vi "PDF_Interface_PDF Protokoll EPA1065_InterferenceVerification.vi"(8 "error in (no error)":errorcluster caption="Fehler (Eingang, kein Fehler)", 11 "Save PDF File Path":path) -> (0 "error out":errorcluster caption="Fehler (Ausgang)")   [LabVIEW 2020, in "EPA 1065.lvlib" / "Interference verificaton 1065-375.lvlib"]
uses:
  Interference verificaton 1065-375.lvlib
  Visualisierungs Elemente/String - Ausgabefeld.ctl
  ResultTable.ctl
  Sprachverwaltung/FGV Aktion Tabelle zerlegen.ctl
  <vilib>/Utility/miscctls.llb/LVRowAndColumnTypeDef.ctl
  Aktion FGV Interference.ctl
  Seiten/FT-IR/FGV FT-IR Aktionen.ctl
  Aktion Index uebersetzten.ctl
  Seiten/System Einstellungen V2/Aktioen FGV System Konstanten.ctl
  PDF_Interface/PDF Protokoll Standard Kopf Optionen.ctl
  <vilib>/Simplicity AI/SAI_PDF_API/Classes/Context/Controls/SAI_PDF_PDF Details.ctl
  PDF_Interface/PDF Interface Helper/PDFContentType.ctl
  PDF_Interface/PDF Interface Helper/PDFTableContentType.ctl
  PDF_Interface/PDF Interface Helper/PDFResults.ctl
  PDF_Interface/PDF Interface Helper/PDFResultPictures.ctl
  PDF_Interface/PDF Interface Helper/PDFCommentPosition.ctl
  PDF_Interface/PDF Interface Helper/PDFPageBreak.ctl
  PDF_Interface/PDF Interface Helper/PDFTablePictures.ctl
  PDF_Interface/PDF Interface Helper/PDFBemerkung.ctl
  <vilib>/Simplicity AI/SAI_PDF_API/Classes/Context/Controls/SAI_PDF_Text Align.ctl
  <vilib>/Simplicity AI/SAI_PDF_API/Classes/Context/Controls/SAI_PDF_Font.ctl
  <vilib>/Simplicity AI/SAI_PDF_API/Classes/Context/Controls/SAI_PDF_Font Encoding.ctl
  Allgemein/allgemeine Sub-VIs.lvlib
  Seiten/FT-IR/Span/Spanfaktor.lvlib
  Seiten/FT-IR/FT-IR.lvlib
  Sprachverwaltung/Sprachverwaltung.lvlib
  Seiten/System Einstellungen V2/System Einstellungen V2.lvlib
  PDF_Interface/PDF Interface.lvlib
  PDF_Interface/PDF Interface Helper/PDF Interface Helper.lvlib
  <vilib>/Simplicity AI/SAI_PDF_API/Classes/Context/Context.lvclass
  Linearisierung V2/Protokoll/Protokoll.lvlib
panel:
  out "[ppm]":sgl=1.0 caption="Grenze:" min=0 format="%#.6g"
  out "[ppm]":sgl=120.0 caption="Querempfindlichkeit:" min=0 format="%#.6g"
  out "LIN Ausgabetabelle":T1
  out "Komponente:":T2 caption="ppm"
  out "ErgebnisTabelle":string[][](table) caption="Tabelle 3"
  out "Header Tabelle":string[][](table) caption="Tabelle"
  # "Interference Verification - EPA § 1065.375"
  # "Ergebnis"
  # "Analysis"
  # "Komponente:"
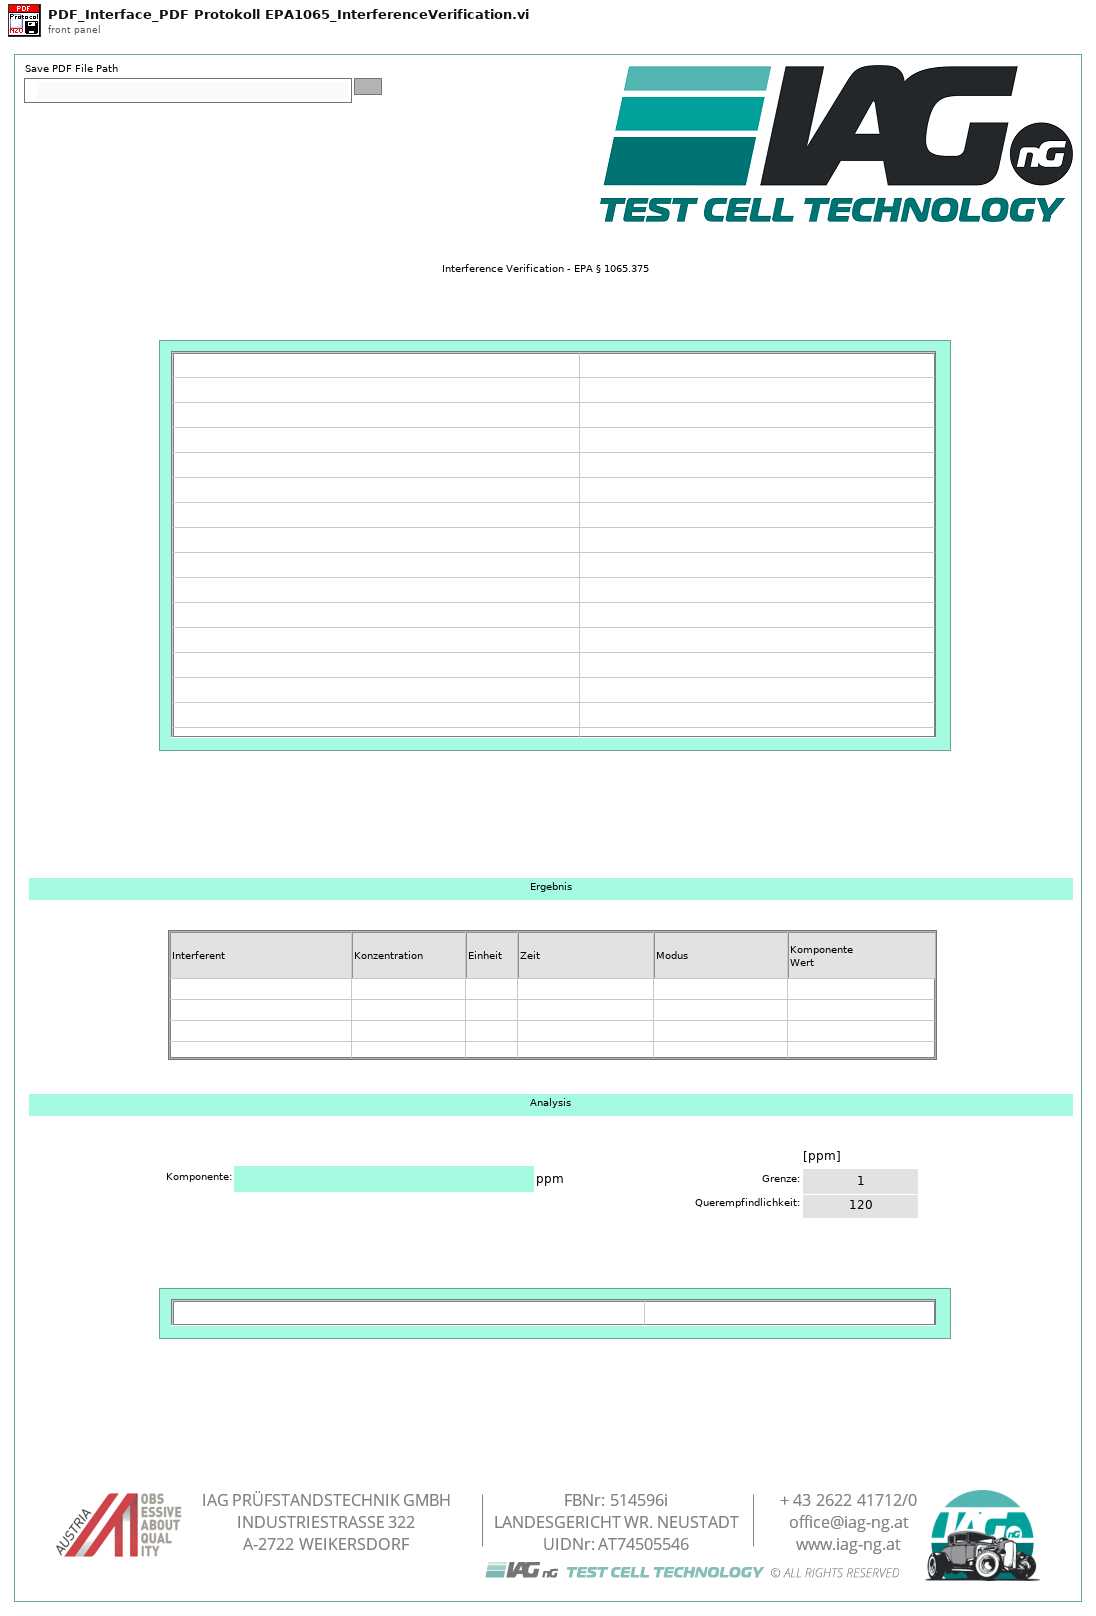
[diagram p1: front panel]
types:
  T1 = typedef "EPA 1065.lvlib/Interference verificaton 1065-375.lvlib/ResultTable.ctl" = string[][]
  T2 = typedef "String - Ausgabefeld.ctl" = string
  T3 = typedef "Sprachverwaltung.lvlib/FGV Aktion Tabelle zerlegen.ctl" = enum16{"laden", "vereinzeln", "speichern"}
  T4 = typedef "PDF Interface.lvlib/PDF Protokoll Standard Kopf Optionen.ctl" = cluster{"Analysator":bool, "FT-IR Rezept":bool, "Gasteiler":bool, "Gas Komponente":bool, "Gas Flasche":bool, "LIN Protokoll":bool, "Operator":bool}
  T5 = typedef "System Einstellungen V2.lvlib/Aktioen FGV System Konstanten.ctl" = enum16{"lesen", "laden", "speichern", "Sprache"}
  T6 = typedef "EPA 1065.lvlib/Interference verificaton 1065-375.lvlib/Aktion Index uebersetzten.ctl" = enum16{"lesen", "schreiben", "auswerten"}
  T7 = typedef "FT-IR.lvlib/FGV FT-IR Aktionen.ctl" = enum16{"lesen", "NOG setzen", "NOS setzen", "Initialisieren", "speichern", "ALLES setzen", "FT-IR Spektrum loggen", "Komm Stoppen", "Spektrum LogKonfig"}
  T8 = typedef "EPA 1065.lvlib/Interference verificaton 1065-375.lvlib/Aktion FGV Interference.ctl" = enum16{"Lesen", "TestKonfig", "TestSetting", "Einheiten", "Ergebnis", "Laden", "Tabelle", "Speichern", "löschen"}
  T9 = typedef "LVRowAndColumnTypeDef.ctl" = cluster{"Row":i32, "Column":i32}
  T10 = typedef "PDF Interface.lvlib/PDF Interface Helper.lvlib/PDFResults.ctl" = cluster{"Results":cluster{"Result Text":string, "Result":bool}[], "ResultPictures":T11, "use Pictures":bool, "Image Scale (%)":sgl, "Autoscale? (T)":bool, "Horizontal Align":i32, "Position":i32}
  T11 = typedef "PDF Interface.lvlib/PDF Interface Helper.lvlib/PDFResultPictures.ctl" = cluster{"Yes Ctl Refnum":refnum<vi>, "No Ctl Refnum":refnum<vi>}
  T12 = typedef "PDF Interface.lvlib/PDF Interface Helper.lvlib/PDFContentType.ctl" = cluster{"Titel":string, "Header Table":string[][], "Table Array":T13[], "Bemerkungen":T17[]}
  T13 = typedef "PDF Interface.lvlib/PDF Interface Helper.lvlib/PDFTableContentType.ctl" = cluster{"TableHeader":string[], "Table":string[][], "Relative Column Widths (%)":sgl[], "Results":T10, "PositionBemerkung":T14, "PageBreak":T15, "TablePictures":T16, "Horizontal Align":i32}
  T14 = typedef "PDF Interface.lvlib/PDF Interface Helper.lvlib/PDFCommentPosition.ctl" = enum16{"before", "after"}
  T15 = typedef "PDF Interface.lvlib/PDF Interface Helper.lvlib/PDFPageBreak.ctl" = enum16{"none", "before", "after", "after comment"}
  T16 = typedef "PDF Interface.lvlib/PDF Interface Helper.lvlib/PDFTablePictures.ctl" = cluster{"Ctl Refnum In":refnum<vi>[], "RowOrColumn":enum16{"Row", "Column"}, "IndexToInsert":u16, "Image Scale (%)":sgl[], "Autoscale? (T)":bool[], "Horizontal Align":i32}
  T17 = typedef "PDF Interface.lvlib/PDF Interface Helper.lvlib/PDFBemerkung.ctl" = cluster{"Bemerkung Text":string, "Align (Left)":T18, "Add Line Feeds (F:No)":bool, "Font":T19}
  T18 = typedef "SAI_PDF_Toolkit.lvlib/Context.lvclass/SAI_PDF_Text Align.ctl" = i32
  T19 = typedef "SAI_PDF_Toolkit.lvlib/Context.lvclass/SAI_PDF_Font.ctl" = cluster{"Font":string, "Size":i32, "Colour":u32, "Bold":bool, "Italic":bool, "Underline":bool, "Strikethrough":bool, "Font Encoding":T20}
  T20 = typedef "SAI_PDF_Toolkit.lvlib/Context.lvclass/SAI_PDF_Font Encoding.ctl" = enum16{"Cp1252, WinANSI", "IdentityH", "IdentityV", "Cp1250", "Cp1257", "MacRoman"}
  T21 = typedef "SAI_PDF_Toolkit.lvlib/Context.lvclass/SAI_PDF_PDF Details.ctl" = cluster{"Title":string, "Subject":string, "Keywords":string, "Author":string, "Creator":string}
  T22 = cluster{"Header Footer Text Cluster":cluster{"Header Text":string, "Footer Text":string, "Time":string, "Page Number":string}, "PDF Details":T21}
  T23 = typedef "EPA 1065.lvlib/Interference verificaton 1065-375.lvlib/TestSetting.ctl" = cluster{"Bearbeiter:":string, "Pfad:":path, "Textname:":string, "Analysator":T24}
  T24 = typedef "System Einstellungen V2.lvlib/Analysatoren.ctl" = string
  T25 = typedef "EPA 1065.lvlib/Interference verificaton 1065-375.lvlib/TestKonfig.ctl" = cluster{"Komponente:":u16, "Modus":T26, "CG Aufschaltzeit:":dbl, "Interferent 1:":u16, "Interferent 2:":u16, "Interferent 3:":u16, "Gasflaschen Nr.:":string, "Gasflaschen Nr.: 2":string, "Gasflaschen Nr.: 3":string, "Inter 1 aktiv":bool, "Inter 2 aktiv":bool, "Inter 3 aktiv":bool, "Accuracy":string, "Accuracy 2":string, "Accuracy 3":string, "Konzentration 1:":dbl, "Konzentration 2:":dbl, "Konzentration 3:":dbl}
  T26 = typedef "EPA 1065.lvlib/Interference verificaton 1065-375.lvlib/Modus.ctl" = u16
  T27 = typedef "EPA 1065.lvlib/Interference verificaton 1065-375.lvlib/Komponenten.ctl" = cluster{"Komponente":T2, "Komponente Index":i32, "Komponente 2":T2, "Komponente Index 2":i32, "Komponente 3":T2, "Komponente Index 3":i32, "Interferent 1":T2, "Interferent Index":i32, "Interferent 2":T2, "Interferent 2 Index":i32, "Interferent 3":T2, "Interferent 3 Index":i32, "Interferent 4":T2, "Interferent 4 Index":i32}
  T28 = cluster{"Modell":string, "ProjektNummer":string, "Software Version":string, "Seriennummer":string}
  T29 = cluster{"Header Size":i32, "Column Ratio left":sgl[]}
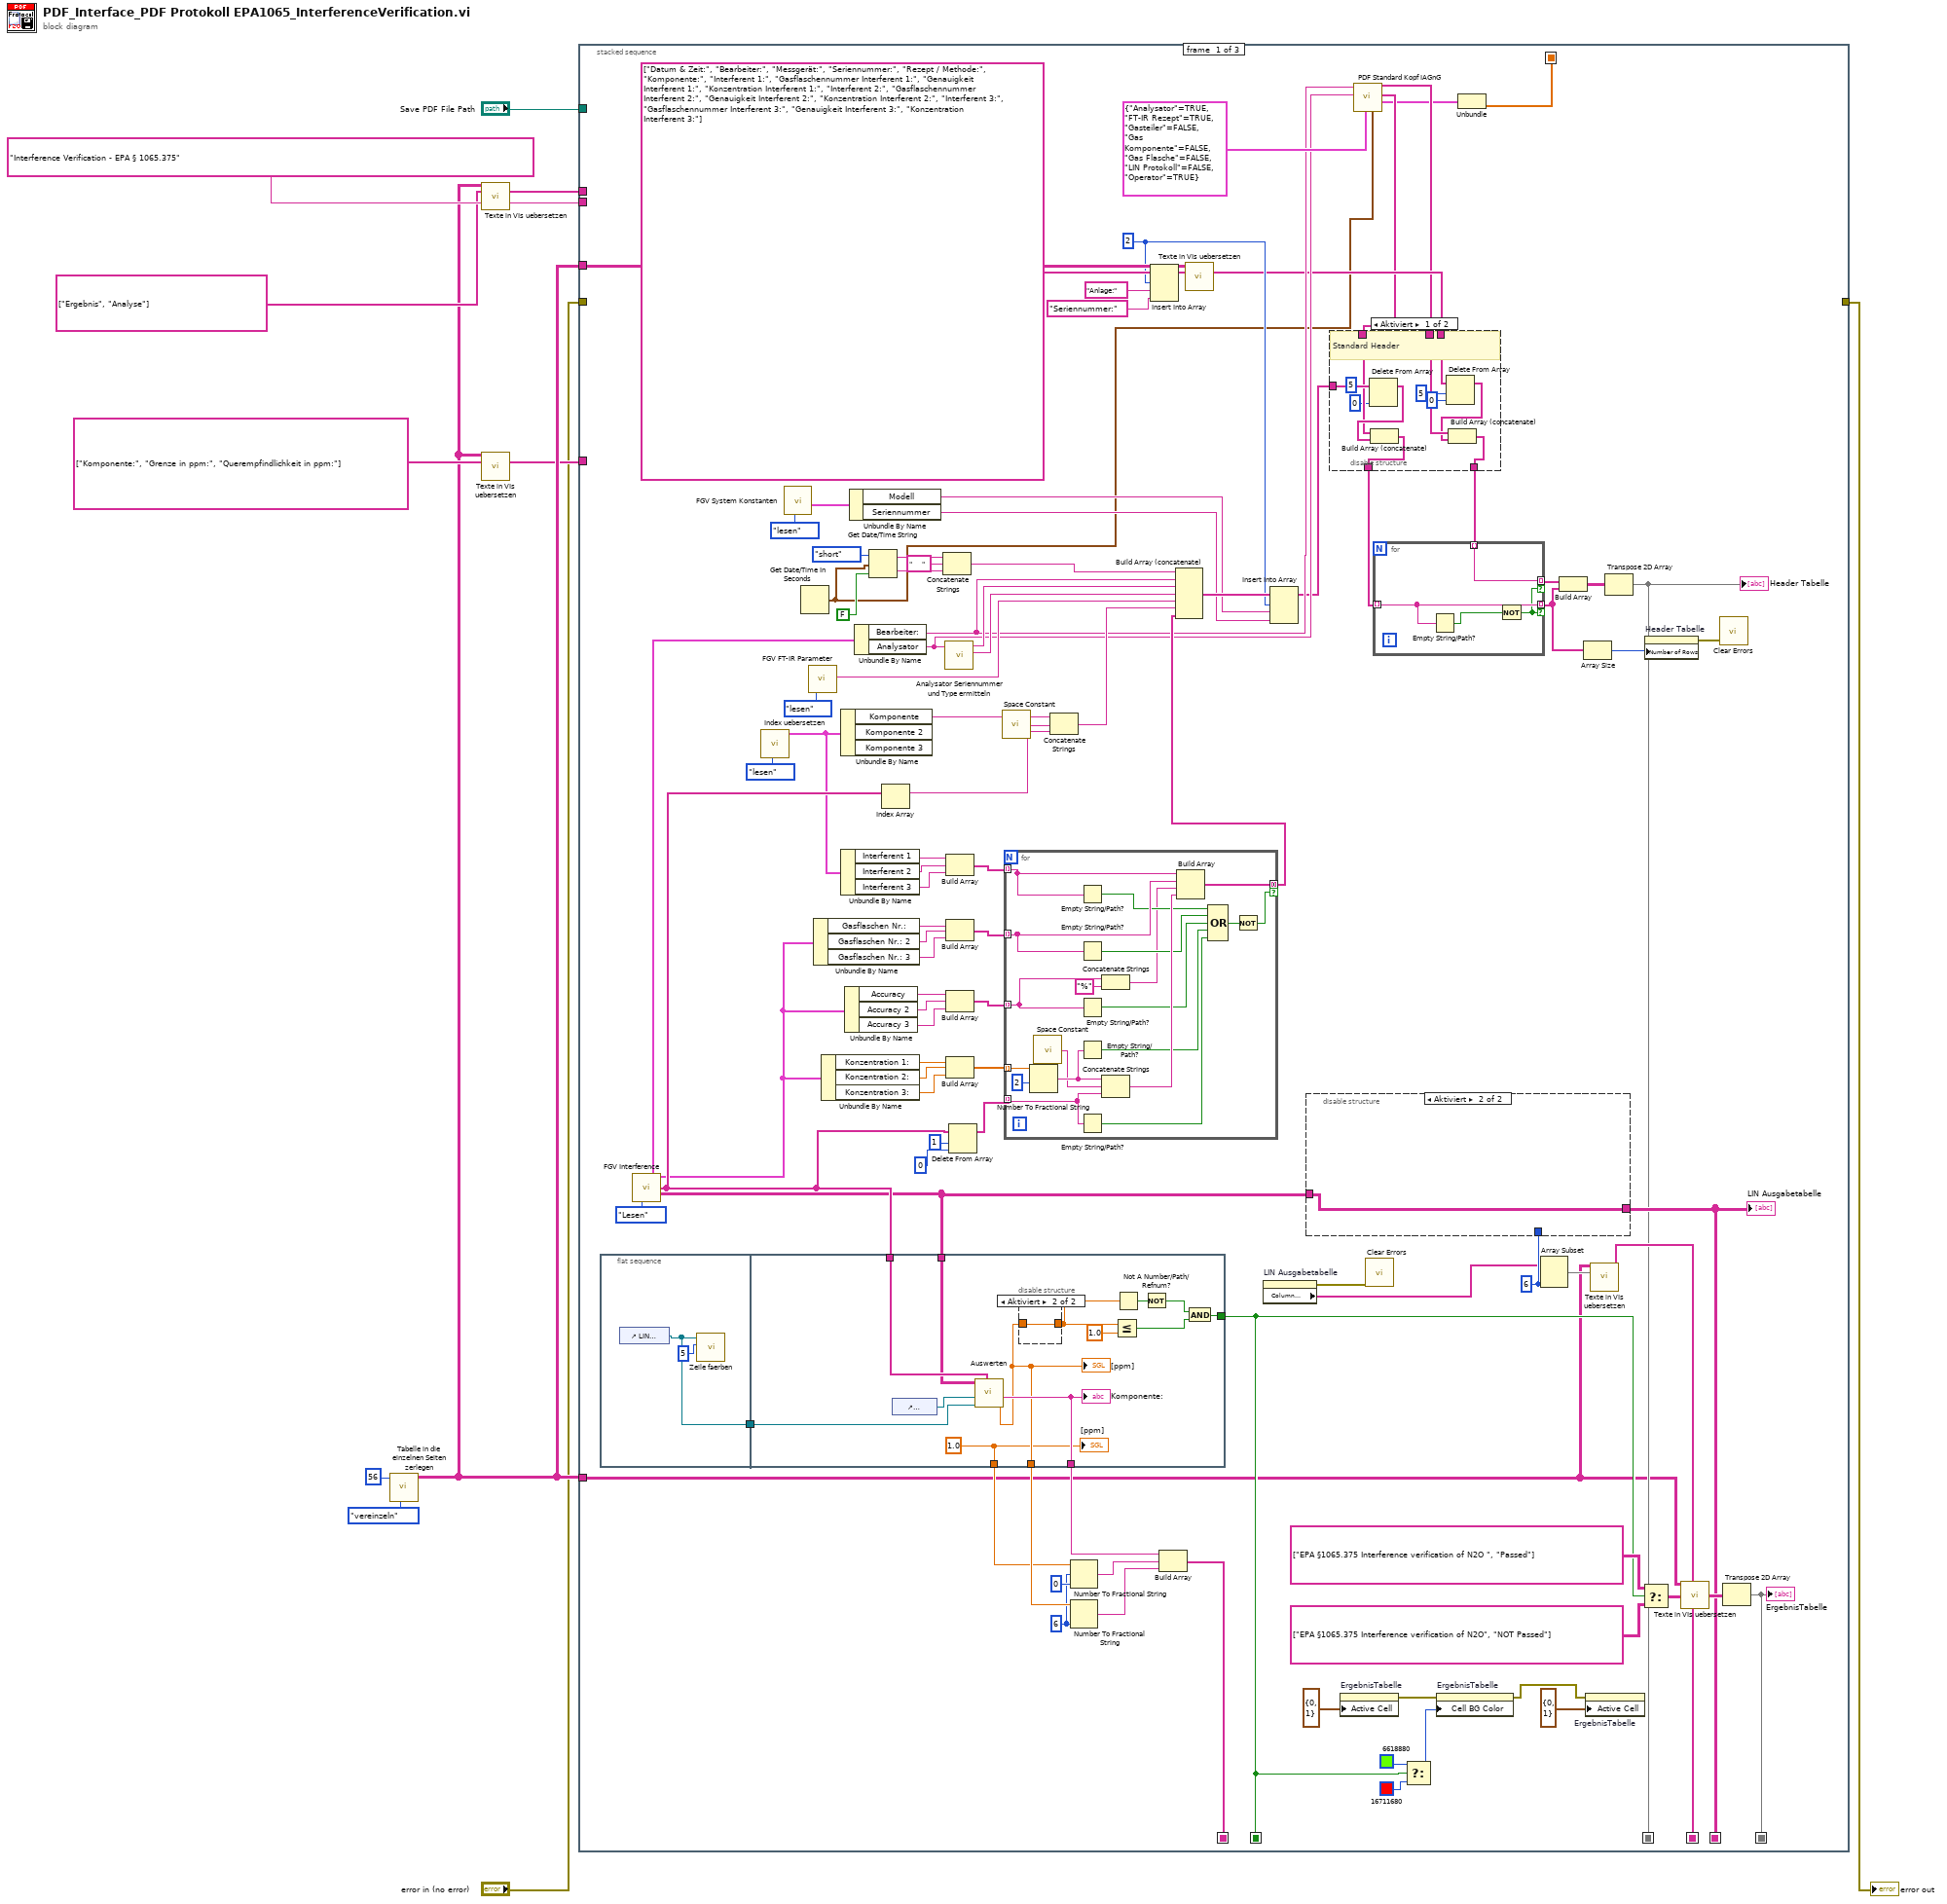
[diagram p0: block diagram]
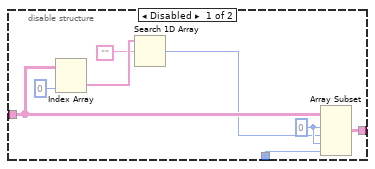
[diagram p2: hidden frame]
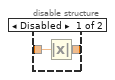
[diagram p4: hidden frame]
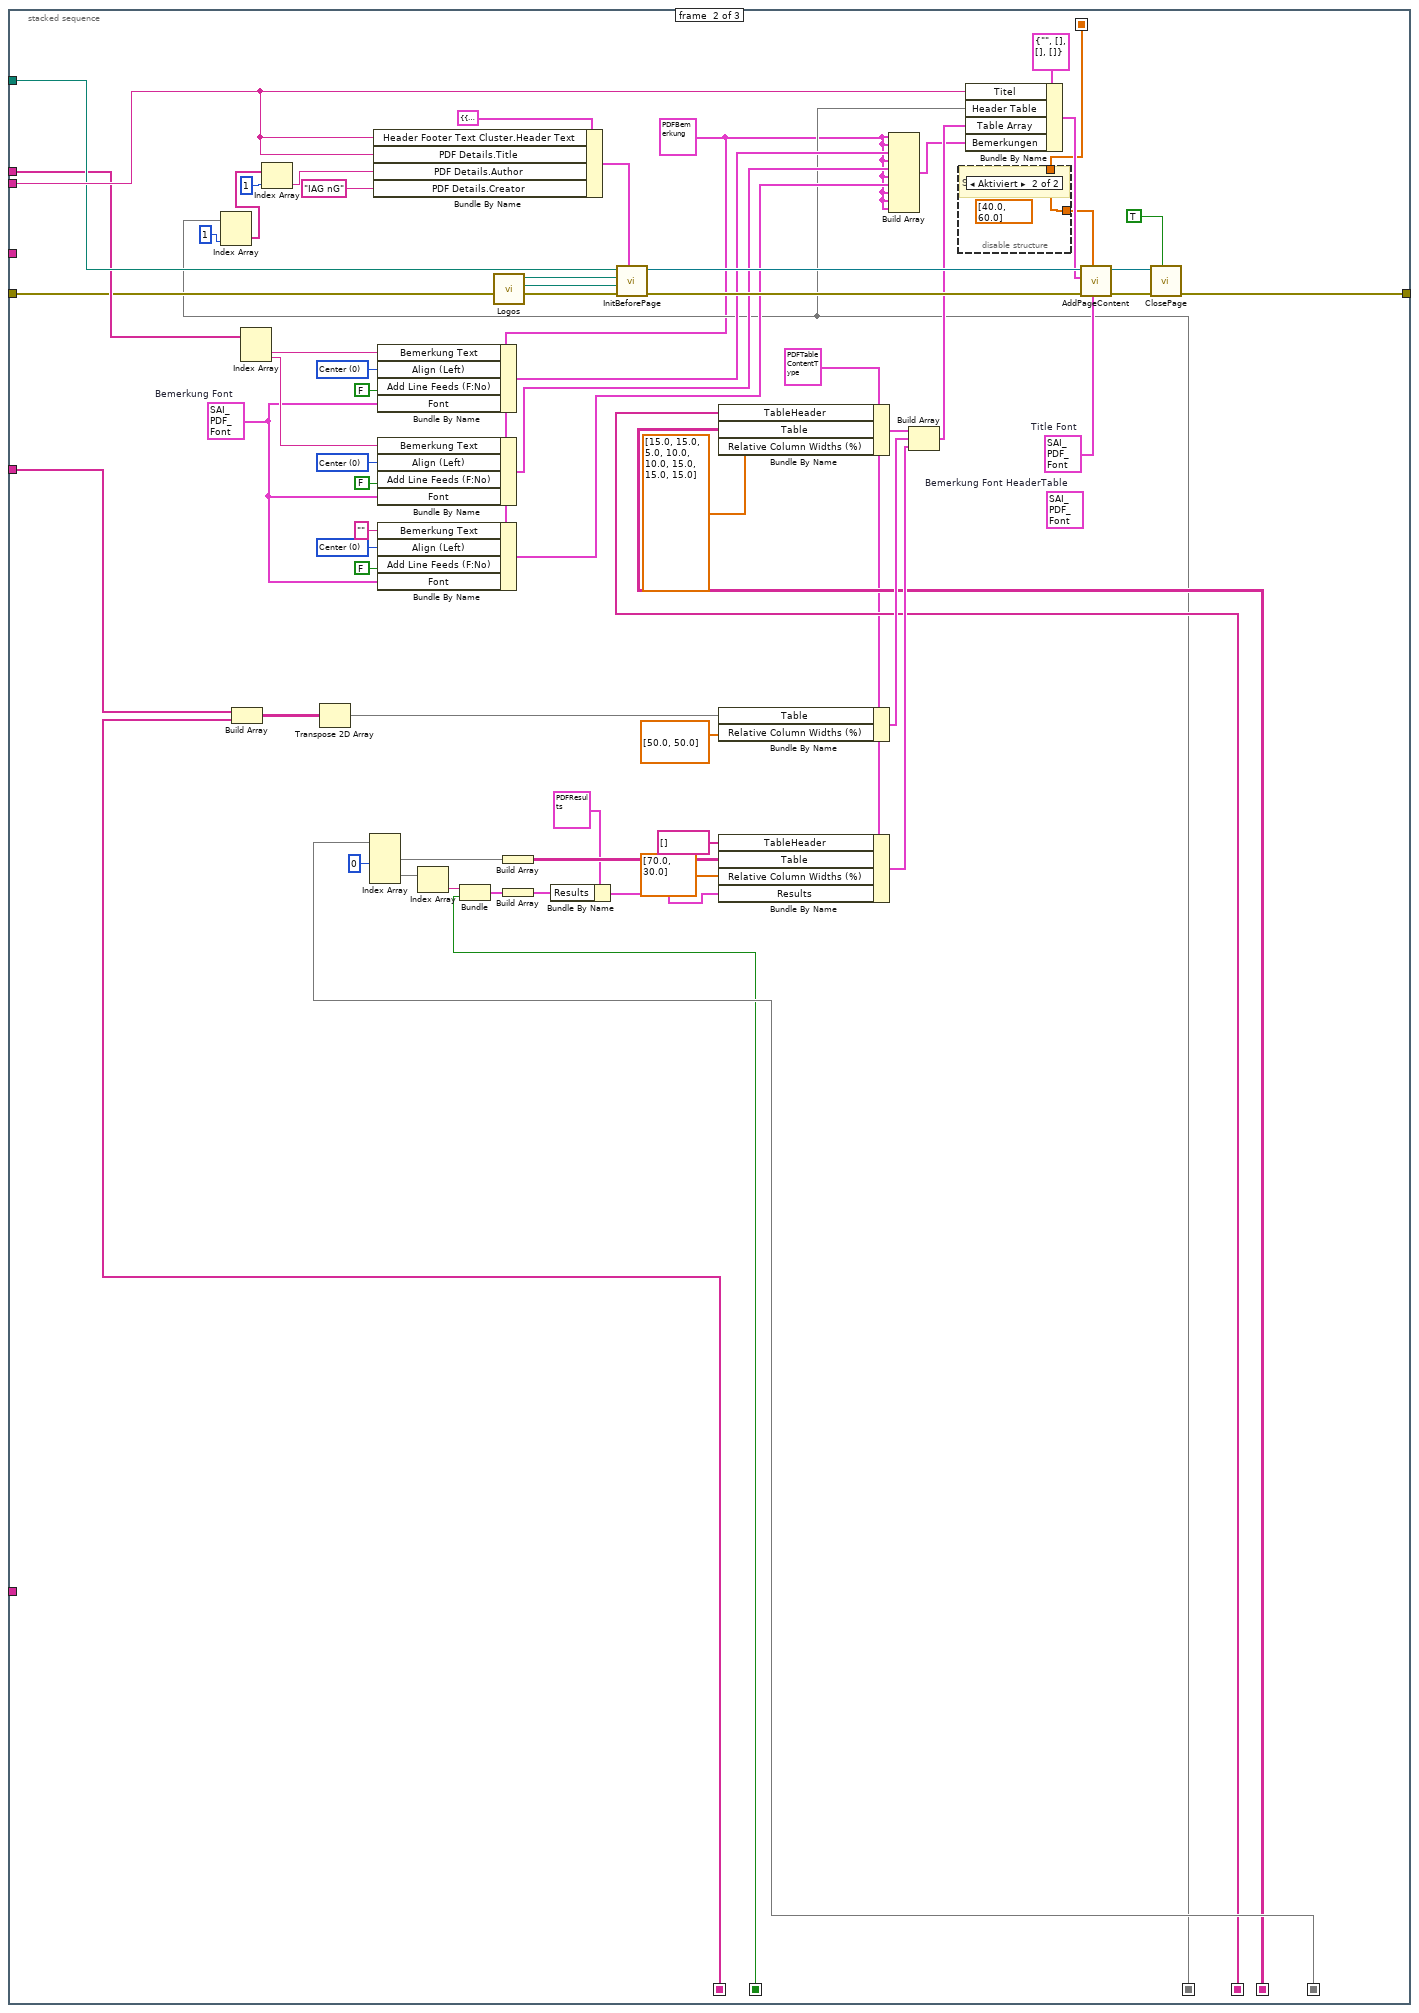
[diagram p5: hidden frame]
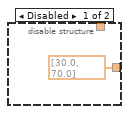
[diagram p6: hidden frame]
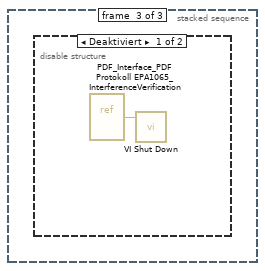
[diagram p7: hidden frame]
diagram:
  n1 = call "Tabelle in die einzelnen Seiten zerlegen.vi"("Aktion"=FGV_Aktion_Tabelle_zerlegen."vereinzeln", "Index (Seite)"=56) -> ("Sprachliste"=w6:string[][])  [unwired: 7 in, 2 out]
  n2 = call "Texte in VIs uebersetzen.vi"("Sprachliste"=w6, "String-Array zum Übersetzen"=string[] ["Ergebnis", "Analyse"], "String zum Übersetzen"="Interference Verification - EPA § 1065.375") -> ("String-Array zum Übersetzen"=w3:string[], "String zum Übersetzen"=w5:string)  [unwired: 8 in, 3 out]
  n3 = call "Texte in VIs uebersetzen.vi"("Sprachliste"=w6, "String-Array zum Übersetzen"=string[] ["Komponente:", "Grenze in ppm:", "Querempfindlichkeit in ppm:"]) -> ("String-Array zum Übersetzen"=w4:string[])  [unwired: 9 in, 4 out]
  n4 = stacked-sequence {
    seq-local: [w45 _ _] -> [_ w186 _]
    seq-local: [w44 _ _] -> [_ w187 _]
    seq-local: [w39 _ _] -> [_ w185 _]
    seq-local: [w38 _ _] -> [_ w184 _]
    seq-local: [w36 _ _] -> [_ w183 _]
    seq-local: [w30 _ _] -> [_ w190 _]
    seq-local: [w13 _ _] -> [_ w176 _]
    tunnel: w6 -> [w29 _ _]
    tunnel: w6 -> [w59 _ _]
    tunnel: "Save PDF File Path" -> [_ w193 _]
    tunnel: w5 -> [_ w194 _]
    tunnel: w4 -> [_ w191 _]
    tunnel: w3 -> [_ w192 _]
    tunnel: "error in (no error)" -> [_ w189 _]
    tunnel: [_ w188 _] -> w1
    frame #0 {
      w32 = i16 6 ("Genauigkeit (6)")
      w41 = 6 ("Länge")
      w46 = 2 ("Index")
      n5 = flat-sequence {
        tunnel: [w158] -> w102
        tunnel: w102 -> [w172]
        tunnel: [w163] -> w45
        tunnel: w84 -> [w169]
        tunnel: w37 -> [w168]
        tunnel: [w162] -> w35
        tunnel: [w161] -> w34
        tunnel: [w160] -> w31
        frame #0 {
          n6 = control-ref of="LIN Ausgabetabelle"() -> (w158:refnum<vi>)
          n7 = call "Zeile faerben.vi"("Anzahl"=5, "Table (Eingang)"=w158) -> ()  [unwired: 9 in, 1 out]
        }
        frame #1 {
          w160 = sgl 1.0 ("[ppm]")
          n8 = control-ref of="Komponente:"() -> (w171:refnum<vi>)
          n9 = call "Auswerten.vi"("Êinheiten"=w169, "LIN Ausgabetabelle"=w172, "Komponente:"=w171, "Tabelle"=w168) -> ("Konzentration Komponente"=w161:dbl, "Komponente:"=w162:T2)  [unwired: 4 in, 2 out]
          "Komponente:" <- w162
          "[ppm]" <- w161
          n10 = disable-structure shown="Aktiviert" {
            disable-tunnel: [w174 w175] -> w167
            disable-tunnel: w161 -> [w173 w175]
            frame Disabled {
              n11 = Absolute Value(x=w173) -> (abs(x)=w174:dbl)
            }
            frame Enabled {
            }
          }
          n12 = Less Or Equal?(x=w167, y=1.0) -> (x <= y?=w165:bool)
          n13 = Not A Number/Path/Refnum?(number/path/refnum=w167) -> (NaN/Path/Refnum?=w166:bool)
          n14 = Not(x=w166) -> (.not. x?=w164:bool)
          n15 = And(x=w164, y=w165) -> (x .and. y?=w163:bool)
          "[ppm]" <- w160
        }
      }
      n16 = call "FGV Interference.vi"("Aktion FGV Interference"=Aktion_FGV_Interference."Lesen") -> ("TestSetting"=w100:T23, "TestKonfig 2"=w66:T25, "Êinheiten"=w84:string[], "Tabelle"=w37:T2[][])  [unwired: 9 in, 2 out]
      n17 = call "Index uebersetzen.vi"("Aktion"=Aktion_Index_uebersetzten."lesen") -> ("Komponenten"=w79:T27)  [unwired: 9 in, 1 out]
      n18 = call "FGV System Konstanten.vi"("Aktionen"=Aktioen_FGV_System_Konstanten."lesen") -> ("Cluster out"=w54:T28)  [unwired: 6 in, 4 out]
      n19 = Get Date/Time In Seconds() -> (seconds since 1Jan1904=w15:timestamp)
      n20 = call "FGV FT-IR Parameter.vi"("Aktion"=FGV_FT-IR_Aktionen."lesen") -> ("Current Recipe"=w90:string)  [unwired: 11 in, 7 out]
      n21 = Unbundle By Name(w66) -> ("Gasflaschen Nr.:"=w78:string, "Gasflaschen Nr.: 2"=w77:string, "Gasflaschen Nr.: 3"=w76:string)
      n22 = Unbundle By Name(w66) -> ("Konzentration 1:"=w75:dbl, "Konzentration 2:"=w74:dbl, "Konzentration 3:"=w73:dbl)
      n23 = Unbundle By Name(w79) -> ("Komponente"=w57:T2)  [unwired: 2 out]
      n24 = Unbundle By Name(w79) -> ("Interferent 1"=w82:T2, "Interferent 2"=w81:T2, "Interferent 3"=w80:T2)
      n25 = Unbundle By Name(w66) -> ("Accuracy"=w65:string, "Accuracy 2"=w64:string, "Accuracy 3"=w63:string)
      n26 = Unbundle By Name(w54) -> ("Modell"=w48:string, "Seriennummer"=w47:string)
      n27 = Unbundle By Name(w100) -> ("Bearbeiter:"=w23:string, "Analysator"=w22:T24)
      n28 = Get Date/Time String(date format (0)=enum16{"short", "long", "abbreviated"}."short" ("Datumsformat (0)"), seconds (now)=w15, want seconds? (F)=FALSE ("Angabe von Sekunden? (F)")) -> (date string=w99:string, time string=w98:string)
      n29 = Index Array(array=w84) -> (element=w56:string)  [unwired: 1 in]
      n30 = Concatenate Strings(w99, "     " ("String"), w98) -> (w92:string)
      n31 = call "Analysator Seriennummer und Type ermitteln.vi"("Analysator"=w22) -> ("Type"=w25:string, "Name für Protokoll"=w26:string)  [unwired: 8 in, 1 out]
      n32 = Build Array(w82, w81, w80) -> (w72:T2[])
      n33 = Build Array(w78, w77, w76) -> (w71:string[])
      n34 = Build Array(w65, w64, w63) -> (w62:string[])
      n35 = Build Array(w75, w74, w73) -> (w70:dbl[])
      n36 = Delete From Array(array=w84, length=1 ("Länge"), index=0 ("Index")) -> (array with subset deleted=w68:string[])  [unwired: 1 out]
      n37 = call <vilib>:"Space Constant.vi"() -> ("String"=w58:string)
      n38 = for {
        tunnel: w72 -> [w150] mode=indexing
        tunnel: w71 -> [w149] mode=indexing
        tunnel: w70 -> [w153] mode=indexing
        tunnel: w68 -> [w152] mode=indexing
        tunnel: [w147] -> w67 mode=concatenating if=w135
        tunnel: w62 -> [w136] mode=indexing
        n39 = Number To Fractional String(number=w153, precision (6)=i16 2 ("Genauigkeit (6)")) -> (F-format string=w151:string)  [unwired: 2 in]
        n40 = call <vilib>:"Space Constant.vi"() -> ("String"=w141:string)
        n41 = Empty String/Path?(string/path=w150) -> (empty?=w146:bool)
        n42 = Empty String/Path?(string/path=w149) -> (empty?=w145:bool)
        n43 = Empty String/Path?(string/path=w136) -> (empty?=w137:bool)
        n44 = Empty String/Path?(string/path=w151) -> (empty?=w142:bool)
        n45 = Empty String/Path?(string/path=w152) -> (empty?=w144:bool)
        n46 = Concatenate Strings(w136, "%" ("String")) -> (w139:string)
        n47 = Concatenate Strings(w151, w141, w152) -> (w148:string)
        n48 = Build Array(w150, w149, w139, w148) -> (w147:T2[])
        n49 = Compound Arithmetic op=OR ("Mehrfacharithmetik")(w146, w145, w137, w142, w144) -> (w143:bool)
        n50 = Not(x=w143) -> (.not. x?=w135:bool)
      }
      n51 = Concatenate Strings(w57, w58, w56) -> (w91:string)
      n52 = Number To Fractional String(number=w31, width (-)=w32, precision (6)=i16 0 ("Genauigkeit (6)")) -> (F-format string=w28:string)  [unwired: 1 in]
      n53 = Number To Fractional String(number=w34, precision (6)=w32) -> (F-format string=w27:string)  [unwired: 2 in]
      n54 = Insert Into Array(array=string[] ["Datum & Zeit:", "Bearbeiter:", "Messgerät:", "Seriennummer:", "Rezept / Methode:", "Komponente:", "Interferent 1:", "Gasflaschennummer Interferent 1:", "Genauigkeit Interferent 1:", "Konzentration Interferent 1:", "Interferent 2:", "Gasflaschennummer Interferent 2:", "Genauigkeit Interferent 2:", "Konzentration Interferent 2:", "Interferent 3:", "Gasflaschennummer Interferent 3:", "Genauigkeit Interferent 3:", "Konzentration Interferent 3:"], index=w46, new element #1="Anlage:" ("Neues Element/Teil-Array"), new element #2="Seriennummer:" ("Neues Element/Teil-Array")) -> (w50:string[])
      n55 = Build Array(w35, w28, w27) -> (w30:T2[])
      n56 = Build Array (concatenate)(w92, w23, w26, w25, w90, w91, w67) -> (w49:T2[])
      n57 = call "Texte in VIs uebersetzen.vi"("Sprachliste"=w59, "String-Array zum Übersetzen"=w50) -> ("String-Array zum Übersetzen"=w20:string[])  [unwired: 9 in, 4 out]
      n58 = property on="LIN Ausgabetabelle" class="Tbl (strikt)"() -> (error out=w43:errorcluster, "Column Headers[]"=w40:string[])  [unwired: 2 in, 1 out]
      n59 = Insert Into Array(array=w49, index=w46, new element #1=w48, new element #2=w47) -> (w17:T2[])
      n60 = disable-structure shown="Aktiviert" {
        disable-tunnel: w41 -> [w119 _]
        disable-tunnel: [w118 w120] -> w39
        disable-tunnel: w37 -> [w114 w120]
        frame Disabled {
          w113 = 0 ("Index")
          n61 = Index Array(array=w114, index (col)=0 ("Deaktivierter Index (Spalte)")) -> (element=w116:T2[])  [unwired: 1 in]
          n62 = Search 1D Array(1D array=w116, element="") -> (index of element=w112:i32)  [unwired: 1 in]
          n63 = Array Subset(array=w114, index (row)=w113, length (row)=w112, index (col)=w113, length (col)=w119) -> (w118:T2[][])
        }
        frame Enabled {
        }
      }
      "LIN Ausgabetabelle" <- w39
      n64 = property on="ErgebnisTabelle" class="Tbl (strikt)"("Active Cell"=T9 {"Row"=0, "Column"=1} ("Aktive Zelle:Aktive Zelle")) -> (error out=w107:errorcluster)  [unwired: 2 in, 1 out]
      n65 = call "PDF Standard Kopf IAGnG.vi"("Zeitstempel"=w15, "Oprtionen Cluster"=T4 {"Analysator"=TRUE, "FT-IR Rezept"=TRUE, "Gasteiler"=FALSE, "Gas Komponente"=FALSE, "Gas Flasche"=FALSE, "LIN Protokoll"=FALSE, "Operator"=TRUE}, "Analysator"=w22, "Bearbeiter/in"=w23) -> ("Size Cluster"=w14:T29, "Header Values"=w18:T2[], "Header Labels"=w19:string[])  [unwired: 4 in, 1 out]
      n66 = disable-structure shown="Aktiviert" {
        disable-tunnel: [w130 w134] -> w21
        disable-tunnel: w20 -> [w132 w134]
        disable-tunnel: w19 -> [w131 _]
        disable-tunnel: w17 -> [w126 w133]
        disable-tunnel: [w123 w133] -> w16
        disable-tunnel: w18 -> [w124 _]
        frame Enabled {
          # "Standard Header"
          n67 = Delete From Array(array=w126, length=5 ("Länge"), index=0 ("Index")) -> (array with subset deleted=w125:T2[])  [unwired: 1 out]
          n68 = Build Array (concatenate)(w124, w125) -> (w123:T2[])
          n69 = Delete From Array(array=w132, length=5 ("Länge"), index=0 ("Index")) -> (array with subset deleted=w129:string[])  [unwired: 1 out]
          n70 = Build Array (concatenate)(w131, w129) -> (w130:string[])
        }
        frame Disabled {
        }
      }
      n71 = call <vilib>:"Clear Errors.vi"("error in (no error)"=w43) -> ()  [unwired: 5 in, 2 out]
      n72 = for {
        tunnel: w16 -> [w157] mode=indexing
        tunnel: [w157] -> w87 mode=indexing if=w154
        tunnel: [w155] -> w89 mode=indexing if=w154
        tunnel: w21 -> [w155] mode=indexing
        n73 = Empty String/Path?(string/path=w157) -> (empty?=w156:bool)
        n74 = Not(x=w156) -> (.not. x?=w154:bool)
      }
      n75 = Select(t=u32 6618880, s=w45, f=u32 16711680) -> (s? t:f=w108:u32)
      n76 = property on="ErgebnisTabelle" class="Tbl (strikt)"(error in=w107, "Cell BG Color"=w108) -> (error out=w103:errorcluster)  [unwired: 1 in, 1 out]
      n77 = Unbundle(w14) -> ("Column Ratio left"=w13:sgl[])  [unwired: 1 out]
      n78 = Array Subset(array=w40, length=w41) -> (w42:string[])  [unwired: 1 in]
      n79 = Build Array(w89, w87) -> (w88:T2[][])
      n80 = Array Size(array=w87) -> (size(s)=w86:i32)
      n81 = property on="ErgebnisTabelle" class="Tbl (strikt)"(error in=w103, "Active Cell"=T9 {"Row"=0, "Column"=1} ("Aktive Zelle:Aktive Zelle")) -> ()  [unwired: 1 in, 2 out]
      n82 = call "Texte in VIs uebersetzen.vi"("Sprachliste"=w29, "String-Array zum Übersetzen"=w42) -> ("String-Array zum Übersetzen"=w38:string[])  [unwired: 9 in, 4 out]
      n83 = Transpose 2D Array(2D array=w88) -> (transposed array=w36:T2[][])
      "Header Tabelle" <- w36
      n84 = Select(t=string[][] [["EPA §1065.375 Interference verification of N2O "], ["Passed"]] ("Tabelle 3"), s=w45, f=string[][] [["EPA §1065.375 Interference verification of N2O"], ["NOT Passed"]] ("Tabelle 3")) -> (s? t:f=w61:string[][])
      n85 = property on="Header Tabelle" class="Tbl (strikt)"("Number of Rows"=w86) -> (error out=w85:errorcluster)  [unwired: 2 in, 1 out]
      n86 = call "Texte in VIs uebersetzen.vi"("Sprachliste"=w29, "2D String-Array zum Übersetzen"=w61) -> ("2D String-Array zum Übersetzen"=w60:string[][])  [unwired: 9 in, 4 out]
      n87 = call <vilib>:"Clear Errors.vi"("error in (no error)"=w85) -> ()  [unwired: 5 in, 2 out]
      n88 = Transpose 2D Array(2D array=w60) -> (transposed array=w44:string[][])
      "ErgebnisTabelle" <- w44
    }
    frame #1 {
      w178 = T17 {"Bemerkung Text"="", "Align (Left)"=0, "Add Line Feeds (F:No)"=FALSE, "Font"={"Font"="Arial", "Size"=10, "Colour"=0, "Bold"=FALSE, "Italic"=FALSE, "Underline"=FALSE, "Strikethrough"=FALSE, "Font Encoding"=enum."Cp1252, WinANSI"}} ("Bemerkung")
      w182 = T13 {"TableHeader"=[], "Table"=[], "Relative Column Widths (%)"=[], "Results"={"Results"=[], "ResultPictures"={"Yes Ctl Refnum"=refnum, "No Ctl Refnum"=refnum}, "use Pictures"=FALSE, "Image Scale (%)"=0.0, "Autoscale? (T)"=FALSE, "Horizontal Align"=0, "Position"=0}, "PositionBemerkung"=enum."before", "PageBreak"=enum."none", "TablePictures"={"Ctl Refnum In"=[], "RowOrColumn"=enum."Row", "IndexToInsert"=0, "Image Scale (%)"=[], "Autoscale? (T)"=[], "Horizontal Align"=0}, "Horizontal Align"=0} ("Table Array")
      w198 = T18 0 items=["Center", "Justified", "Justified All", "Left", "Right"] ("Align (Left)")
      w218 = T18 0 items=["Center", "Justified", "Justified All", "Left", "Right"] ("Align (Left)")
      w221 = T18 0 items=["Center", "Justified", "Justified All", "Left", "Right"] ("Align (Left)")
      (unwired) T19 {"Font"="Arial", "Size"=12, "Colour"=16711680, "Bold"=TRUE, "Italic"=TRUE, "Underline"=FALSE, "Strikethrough"=FALSE, "Font Encoding"=enum."Cp1252, WinANSI"}  # Bemerkung Font HeaderTable
      w177 = T19 {"Font"="Arial", "Size"=12, "Colour"=0, "Bold"=TRUE, "Italic"=TRUE, "Underline"=FALSE, "Strikethrough"=FALSE, "Font Encoding"=enum."Cp1252, WinANSI"}  # Bemerkung Font
      w227 = T19 {"Font"="Arial", "Size"=24, "Colour"=0, "Bold"=TRUE, "Italic"=FALSE, "Underline"=TRUE, "Strikethrough"=FALSE, "Font Encoding"=enum."Cp1252, WinANSI"}  # Title Font
      n89 = Index Array(array=w183, index (col)=1 ("Index")) -> (element=w214:T2[])  [unwired: 1 in]
      n90 = Build Array(w191, w190) -> (w211:T2[][])
      n91 = Index Array(array=w192) -> (element #1=w196:string, element #2=w200:string)  [unwired: 2 in]
      n92 = Index Array(array=w214, index=1 ("Index")) -> (element=w224:T2)
      n93 = Transpose 2D Array(2D array=w211) -> (transposed array=w201:T2[][])
      n94 = Index Array(array=w187, index (col) #1=0 ("Deaktivierter Index (Spalte)")) -> (element #1=w203:string[], element #2=w206:string[])  [unwired: 3 in]
      n95 = Bundle By Name(cluster=T22 {"Header Footer Text Cluster"={"Header Text"="Protokoll XYZ", "Footer Text"="IAG nG", "Time"="<TIMESTAMP yyyy-MM-dd>", "Page Number"="Page <P> of <PT>"}, "PDF Details"={"Title"="Test PDF", "Subject"="Versa Tabasco", "Keywords"="", "Author"="RIW", "Creator"="IAG"}} ("Info"), "Header Footer Text Cluster.Header Text"=w194, "PDF Details.Title"=w194, "PDF Details.Author"=w224, "PDF Details.Creator"="IAG nG") -> (w232:T22)
      n96 = Bundle By Name(cluster=w178, "Bemerkung Text"=w196, "Align (Left)"=w198, "Add Line Feeds (F:No)"=FALSE, "Font"=w177) -> (w197:T17)
      n97 = Bundle By Name(cluster=w178, "Bemerkung Text"=w200, "Align (Left)"=w221, "Add Line Feeds (F:No)"=FALSE, "Font"=w177) -> (w217:T17)
      n98 = Bundle By Name(cluster=w178, "Bemerkung Text"="", "Align (Left)"=w218, "Add Line Feeds (F:No)"=FALSE, "Font"=w177) -> (w216:T17)
      n99 = Index Array(array=w206) -> (element=w205:string)  [unwired: 1 in]
      n100 = Bundle(w205, w186) -> (w204:cluster{string, bool})  [unwired: 1 in]
      n101 = call "Logos.vi"() -> ("Footer Image File Path"=w240:path, "Header Image File Path"=w241:path)  [unwired: 8 in, 2 out]
      n102 = Build Array(w203) -> (w202:string[][])
      n103 = Build Array(w204) -> (w181:cluster{string, bool}[])
      n104 = Bundle By Name(cluster=T10 {"Results"=[], "ResultPictures"={"Yes Ctl Refnum"=refnum, "No Ctl Refnum"=refnum}, "use Pictures"=FALSE, "Image Scale (%)"=100.0, "Autoscale? (T)"=TRUE, "Horizontal Align"=3, "Position"=0} ("Results"), "Results"=w181) -> (w180:T10)
      n105 = call "InitBeforePage.vi"("Info"=w232, "Fehler (Eingang, kein Fehler)"=w189, "Footer Image File Path"=w240, "Header Image File Path"=w241, "Path (Dialog if Empty)"=w193) -> ("Fehler (Ausgang)"=w239:errorcluster, "Context (Ausgang)"=w238:refnum<class "Context.lvclass">)  [unwired: 5 in]
      n106 = Bundle By Name(cluster=w182, "TableHeader"=w184, "Table"=w185, "Relative Column Widths (%)"=sgl[] [15.0, 15.0, 5.0, 10.0, 10.0, 15.0, 15.0, 15.0]) -> (w226:T13)
      n107 = Bundle By Name(cluster=w182, "Table"=w201, "Relative Column Widths (%)"=sgl[] [50.0, 50.0]) -> (w212:T13)
      n108 = Bundle By Name(cluster=w182, "TableHeader"=string[] [], "Table"=w202, "Relative Column Widths (%)"=sgl[] [70.0, 30.0], "Results"=w180) -> (w213:T13)
      n109 = Build Array(w178, w178, w197, w178, w217, w178, w216, w178, w178, w178) -> (w222:T17[])
      n110 = Build Array(w226, w212, w213) -> (w230:T13[])
      n111 = disable-structure shown="Aktiviert" {
        disable-tunnel: [sgl[] [30.0, 70.0] ("Column Ratio left") w243] -> w228
        disable-tunnel: w176 -> [_ w243]
        frame Disabled {
        }
        frame Enabled {
          (unwired) sgl[] [40.0, 60.0] ("Column Ratio left")
          # "Standard Header"
        }
      }
      n112 = Bundle By Name(cluster=T12 {"Titel"="", "Header Table"=[], "Table Array"=[], "Bemerkungen"=[]} ("Content"), "Titel"=w194, "Header Table"=w183, "Table Array"=w230, "Bemerkungen"=w222) -> (w229:T12)
      n113 = call "AddPageContent.vi"("Title Font"=w227, "Column Ratio left"=w228, "error in"=w239, "Content"=w229, "Context (Eingang)"=w238) -> ("error out"=w237:errorcluster, "Context (Ausgang)"=w236:refnum<class "Context.lvclass">)  [unwired: 5 in]
      n114 = call "ClosePage.vi"("popup viewer"=TRUE, "Fehler (Eingang, kein Fehler)"=w237, "Context (Eingang)"=w236) -> ("Fehler (Ausgang)"=w188:errorcluster)  [unwired: 8 in]
    }
    frame #2 {
      n115 = disable-structure shown="Deaktiviert" {
        frame Disabled {
          n116 = vi-ref "PDF_Interface_PDF Protokoll EPA1065_InterferenceVerification.vi"() -> (w244:refnum<vi>)
          n117 = call "VI Shut Down.vi"("VI Referenz"=w244) -> ()  [unwired: 11 in]
        }
        frame Enabled {
        }
      }
    }
  }
  "error out" <- w1
